vi "high_limit_parser.vi"(1 "Higher limit":dbl=60.0 format="%#_13g", 2 "Delay in":dbl) -> (6 "Delay out":dbl)   [LabVIEW 2015]
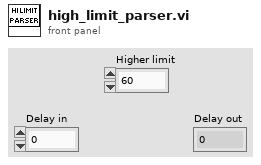
[diagram p1: front panel]
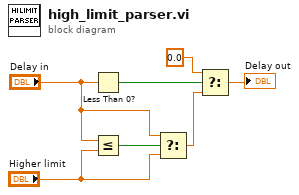
[diagram p0: block diagram]
diagram:
  n1 = Less Than 0?(x="Delay in") -> (x < 0?=w7:bool)
  n2 = Less Or Equal?(x="Delay in", y="Higher limit") -> (x <= y?=w4:bool)
  n3 = Select(t="Delay in", s=w4, f="Higher limit") -> (s? t:f=w5:dbl)
  n4 = Select(t=0.0, s=w7, f=w5) -> (s? t:f=→"Delay out":dbl)
